vi "Create Client Message Queue.vi"(8 "error in (no error)":errorcluster) -> (0 "error out":errorcluster, 3 "Client Message Queues":T1)   [LabVIEW 2024, in "Message Queue.lvlib"]
doc: "Creates and initializes the client message queues for your application. If your application requires more message queues, right-click the Client Message Queues constant above and select Open Type Def. Add the new message queues to the type definition, then initialize them in this VI."
uses:
  Message Queue.lvlib
  Client Message Queues.ctl
  Message Cluster.ctl
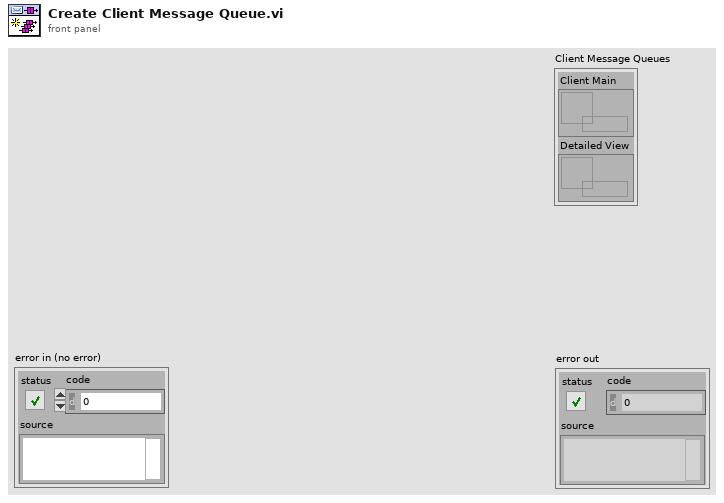
[diagram p1: front panel]
types:
  T1 = typedef "Message Queue.lvlib/Client Message Queues.ctl" = cluster{"Client Main":refnum<queue>, "Detailed View":refnum<queue>}
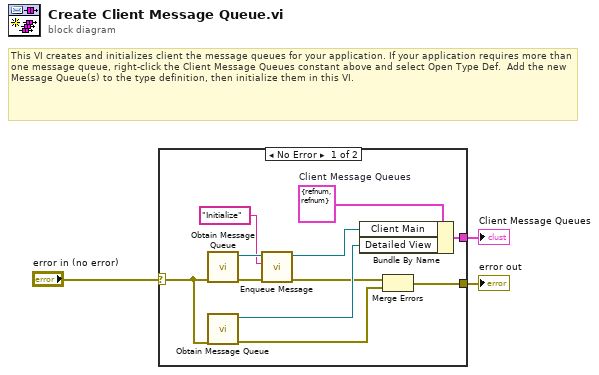
[diagram p0: block diagram]
diagram:
  # "This VI creates and initializes client the message queues for your application. If your application requires more than one message queue, right-click the Client Message Queues constant above and select Open Type Def.  Add the new Message Queue(s) to the type definition, then initialize them in this VI."
  n1 = case shown="No Error" "error in (no error)" {
    selector: "error in (no error)" -> [w4 w15]
    tunnel: [w10 w15] -> w3
    tunnel: [w13 _] -> w1
    frame No Error {
      w12 = T1 {"Client Main"=refnum, "Detailed View"=refnum}  # Client Message Queues
      n2 = call "Obtain Message Queue.vi"("error in (no error)"=w4) -> ("error out"=w9:errorcluster, "Message Queue"=w8:refnum<queue>)  [unwired: 9 in]
      n3 = call "Obtain Message Queue.vi"("error in (no error)"=w4) -> ("error out"=w11:errorcluster, "Message Queue"=w14:refnum<queue>)  [unwired: 9 in]
      n4 = call "Enqueue Message.vi"("error in (no error)"=w9, "Message"="Initialize", "Message Queue"=w8) -> ("error out"=w6:errorcluster, "dup Message Queue"=w7:refnum<queue>)  [unwired: 7 in]
      n5 = Bundle By Name(cluster=w12, "Client Main"=w7, "Detailed View"=w14) -> (w13:T1)
      n6 = Merge Errors(w6, w11) -> (w10:errorcluster)
    }
    frame Error {
    }
  }
  "error out" <- w3
  "Client Message Queues" <- w1
